vi "ni5660 Sub Temperature Adjust Correction.vi"(9 "correction":T1 {"spectrum correction"."correction factors" format="%.2f"; "spectrum correction"."df" format="%.2f"; "spectrum correction"."f0" format="%.2f"}, 10 "temperature correction units":T2(ring)=enum."W", 11 "temperature correction factor":dbl format="%.2f") -> (2 "temperature adjusted correction":T1 {"spectrum correction"."correction factors" format="%.2f"; "spectrum correction"."df" format="%.2f"; "spectrum correction"."f0" format="%.2f"})   [LabVIEW 2011]
doc: "This subVI is used to correct the calibration correction factors of the PXI-5660 RFSA for temperature variations in the RFSA hardware."
uses:
  <vilib>/addons/Spectral Measurements Toolset/LVSupport/SMT niScope Utilities/smt_correction.ctl
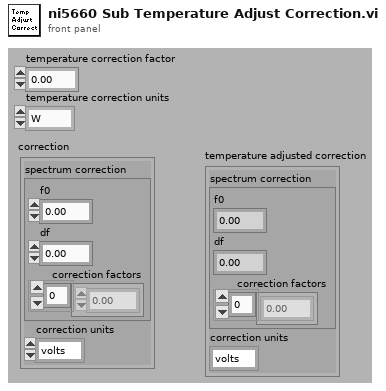
[diagram p1: front panel]
types:
  T1 = typedef "smt_correction.ctl" = cluster{"spectrum correction":cluster{"f0":dbl, "df":dbl, "correction factors":dbl[]}, "correction units":enum16{"volts", "watts", "dB"}}
  T2 = enum16{"V", "V^2", "W", "dBm", "dBW", "dBV", "dBmV", "dBuV"}
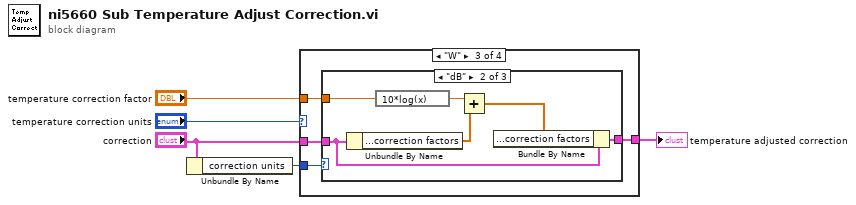
[diagram p0: block diagram]
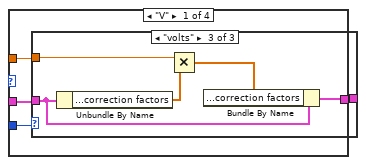
[diagram p2: hidden frame]
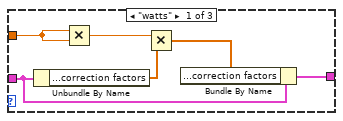
[diagram p3: hidden frame]
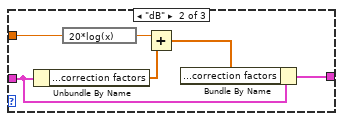
[diagram p4: hidden frame]
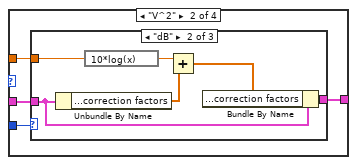
[diagram p5: hidden frame]
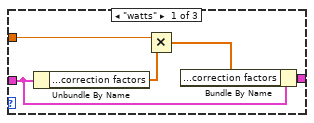
[diagram p6: hidden frame]
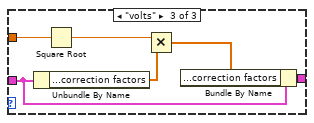
[diagram p7: hidden frame]
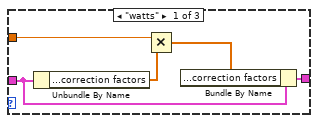
[diagram p8: hidden frame]
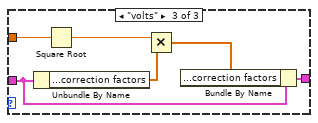
[diagram p9: hidden frame]
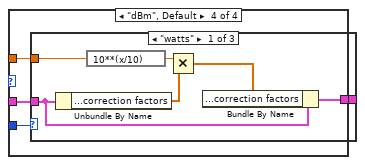
[diagram p10: hidden frame]
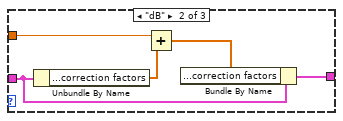
[diagram p11: hidden frame]
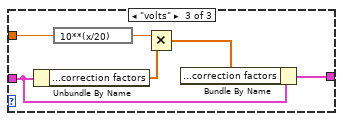
[diagram p12: hidden frame]
diagram:
  n1 = Unbundle By Name("correction") -> ("correction units"=w2:enum16{"volts", "watts", "dB"})
  n2 = case shown="\"W\"" "temperature correction units" {
    tunnel: "correction" -> [w7 w30 w51 w72]
    tunnel: "temperature correction factor" -> [w9 w29 w50 w71]
    tunnel: [w6 w28 w49 w70] -> w3
    tunnel: w2 -> [w8 w27 w48 w69]
    frame "V" {
      n3 = case shown="\"volts\"" w8 {
        tunnel: w7 -> [w14 w19 w25]
        tunnel: w9 -> [w10 w21 w22]
        tunnel: [w12 w17 w23] -> w6
        frame "watts" {
          n4 = Unbundle By Name(w14) -> ("spectrum correction.correction factors"=w15:dbl[])
          n5 = Multiply(x=w10, y=w10) -> (x*y=w11:dbl)
          n6 = Multiply(x=w11, y=w15) -> (x*y=w13:dbl[])
          n7 = Bundle By Name(cluster=w14, "spectrum correction.correction factors"=w13) -> (w12:T1)
        }
        frame "dB" {
          n8 = Unbundle By Name(w19) -> ("spectrum correction.correction factors"=w20:dbl[])
          n9 = expression code="20*log(x)"(w21) -> (w16:dbl)
          n10 = Add(x=w16, y=w20) -> (x+y=w18:dbl[])
          n11 = Bundle By Name(cluster=w19, "spectrum correction.correction factors"=w18) -> (w17:T1)
        }
        frame "volts" {
          n12 = Unbundle By Name(w25) -> ("spectrum correction.correction factors"=w26:dbl[])
          n13 = Multiply(x=w22, y=w26) -> (x*y=w24:dbl[])
          n14 = Bundle By Name(cluster=w25, "spectrum correction.correction factors"=w24) -> (w23:T1)
        }
      }
    }
    frame "V^2" {
      n15 = case shown="\"dB\"" w27 {
        tunnel: w30 -> [w33 w39 w46]
        tunnel: w29 -> [w35 w41 w43]
        tunnel: [w31 w37 w44] -> w28
        frame "watts" {
          n16 = Unbundle By Name(w33) -> ("spectrum correction.correction factors"=w34:dbl[])
          n17 = Multiply(x=w35, y=w34) -> (x*y=w32:dbl[])
          n18 = Bundle By Name(cluster=w33, "spectrum correction.correction factors"=w32) -> (w31:T1)
        }
        frame "dB" {
          n19 = Unbundle By Name(w39) -> ("spectrum correction.correction factors"=w40:dbl[])
          n20 = expression code="10*log(x)"(w41) -> (w36:dbl)
          n21 = Add(x=w36, y=w40) -> (x+y=w38:dbl[])
          n22 = Bundle By Name(cluster=w39, "spectrum correction.correction factors"=w38) -> (w37:T1)
        }
        frame "volts" {
          n23 = Unbundle By Name(w46) -> ("spectrum correction.correction factors"=w47:dbl[])
          n24 = Square Root(x=w43) -> (sqrt(x)=w42:dbl)
          n25 = Multiply(x=w42, y=w47) -> (x*y=w45:dbl[])
          n26 = Bundle By Name(cluster=w46, "spectrum correction.correction factors"=w45) -> (w44:T1)
        }
      }
    }
    frame "W" {
      n27 = case shown="\"dB\"" w48 {
        tunnel: w51 -> [w54 w60 w67]
        tunnel: w50 -> [w56 w62 w64]
        tunnel: [w52 w58 w65] -> w49
        frame "watts" {
          n28 = Unbundle By Name(w54) -> ("spectrum correction.correction factors"=w55:dbl[])
          n29 = Multiply(x=w56, y=w55) -> (x*y=w53:dbl[])
          n30 = Bundle By Name(cluster=w54, "spectrum correction.correction factors"=w53) -> (w52:T1)
        }
        frame "dB" {
          n31 = Unbundle By Name(w60) -> ("spectrum correction.correction factors"=w61:dbl[])
          n32 = expression code="10*log(x)"(w62) -> (w57:dbl)
          n33 = Add(x=w57, y=w61) -> (x+y=w59:dbl[])
          n34 = Bundle By Name(cluster=w60, "spectrum correction.correction factors"=w59) -> (w58:T1)
        }
        frame "volts" {
          n35 = Unbundle By Name(w67) -> ("spectrum correction.correction factors"=w68:dbl[])
          n36 = Square Root(x=w64) -> (sqrt(x)=w63:dbl)
          n37 = Multiply(x=w63, y=w68) -> (x*y=w66:dbl[])
          n38 = Bundle By Name(cluster=w67, "spectrum correction.correction factors"=w66) -> (w65:T1)
        }
      }
    }
    frame "dBm", Default {
      n39 = case shown="\"watts\"" w69 {
        tunnel: w72 -> [w76 w82 w88]
        tunnel: w71 -> [w78 w79 w85]
        tunnel: [w74 w80 w86] -> w70
        frame "watts" {
          n40 = Unbundle By Name(w76) -> ("spectrum correction.correction factors"=w77:dbl[])
          n41 = expression code="10**(x/10)"(w78) -> (w73:dbl)
          n42 = Multiply(x=w73, y=w77) -> (x*y=w75:dbl[])
          n43 = Bundle By Name(cluster=w76, "spectrum correction.correction factors"=w75) -> (w74:T1)
        }
        frame "dB" {
          n44 = Unbundle By Name(w82) -> ("spectrum correction.correction factors"=w83:dbl[])
          n45 = Add(x=w79, y=w83) -> (x+y=w81:dbl[])
          n46 = Bundle By Name(cluster=w82, "spectrum correction.correction factors"=w81) -> (w80:T1)
        }
        frame "volts" {
          n47 = Unbundle By Name(w88) -> ("spectrum correction.correction factors"=w89:dbl[])
          n48 = expression code="10**(x/20)"(w85) -> (w84:dbl)
          n49 = Multiply(x=w84, y=w89) -> (x*y=w87:dbl[])
          n50 = Bundle By Name(cluster=w88, "spectrum correction.correction factors"=w87) -> (w86:T1)
        }
      }
    }
  }
  "temperature adjusted correction" <- w3
